vi "e.gate ASCII Write Value - CORE.vi"(6 "Value":dbl, 8 "error in (no error)":errorcluster, 9 "Boolean":bool=TRUE, 10 "Channel":i32, 11 "e.gate Configuration In":T1) -> (0 "error out":errorcluster, 3 "e.gate Configuration Out":T1)   [LabVIEW 2016]
doc: "<B>AMC - Analytik & Messtechnik GmbH Chemnitz</B>\n\nLabVIEW Drivers for e.gate / e.pac series from Gantner Instruments\n\nThis VI writes a value specified by <B>Channel</B> to a device specified by <B>connection ID In</B>."
uses:
  e.gate Configuration.ctl
  e.gate Channel Data.ctl
  e.gate Data Type.ctl
  e.gate Protocol Type.ctl
  e.gate Module  Data.ctl
  e.gateHSP_DLLhandle.ctl
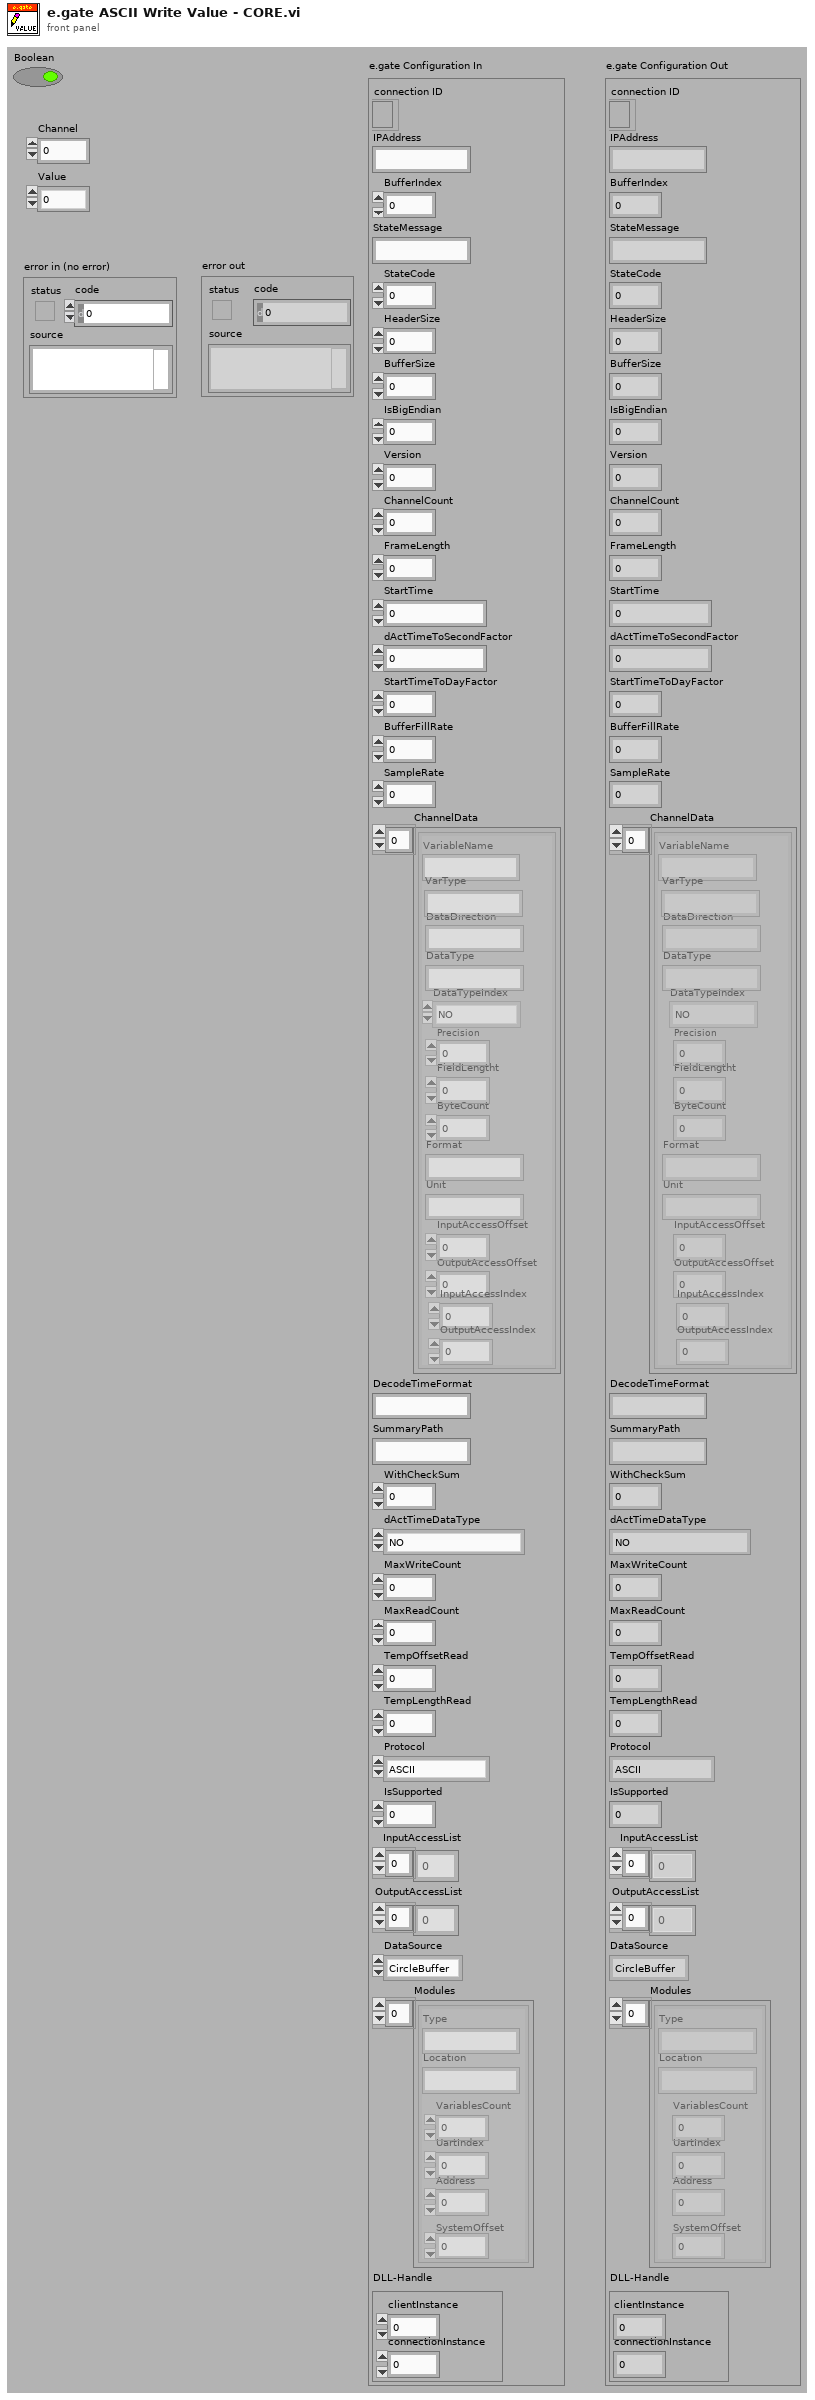
[diagram p1: front panel]
types:
  T1 = typedef "e.gate Configuration.ctl" = cluster{"connection ID":refnum<k5>, "IPAddress":string, "BufferIndex":i32, "StateMessage":string, "StateCode":i8, "HeaderSize":i32, "BufferSize":i32, "IsBigEndian":i32, "Version":i32, "ChannelCount":i32, "FrameLength":i32, "StartTime":dbl, "dActTimeToSecondFactor":dbl, "StartTimeToDayFactor":dbl, "BufferFillRate":dbl, "SampleRate":dbl, "ChannelData":T2[], "DecodeTimeFormat":string, "SummaryPath":string, "WithCheckSum":i32, "dActTimeDataType":T3, "MaxWriteCount":i32, "MaxReadCount":i32, "TempOffsetRead":i32, "TempLengthRead":i32, "Protocol":T4, "IsSupported":i32, "InputAccessList":i32[], "OutputAccessList":i32[], "DataSource":enum16{"CircleBuffer", "test.con Logger", "test.con Archive"}, "Modules":T5[], "DLL-Handle":T6}
  T2 = typedef "e.gate Channel Data.ctl" = cluster{"VariableName":string, "DataDirection":string, "DataType":string, "DataTypeIndex":T3, "Precision":i16, "FieldLengtht":i16, "ByteCount":i32, "Format":string, "Unit":string, "InputAccessOffset":i32, "OutputAccessOffset":i16, "InputAccessIndex":i16, "OutputAccessIndex":i16, "VarType":string}
  T3 = typedef "e.gate Data Type.ctl" = enum16{"NO", "BOOL", "SINT8", "USINT8", "SINT16", "USINT16", "SINT32", "USINT32", "FLOAT", "SET8", "SET16", "SET32", "DOUBLE", "SINT64", "USINT64", "SET64"}
  T4 = typedef "e.gate Protocol Type.ctl" = enum16{"ASCII", "HighspeedPort Online", "HighspeedPort Buffer", "eGateHighspeedPortDLL "}
  T5 = typedef "e.gate Module  Data.ctl" = cluster{"Type":string, "Location":string, "VariablesCount":i16, "UartIndex":i16, "Address":i16, "SystemOffset":i16}
  T6 = typedef "e.gateHSP_DLLhandle.ctl" = cluster{"clientInstance":i32, "connectionInstance":i32}
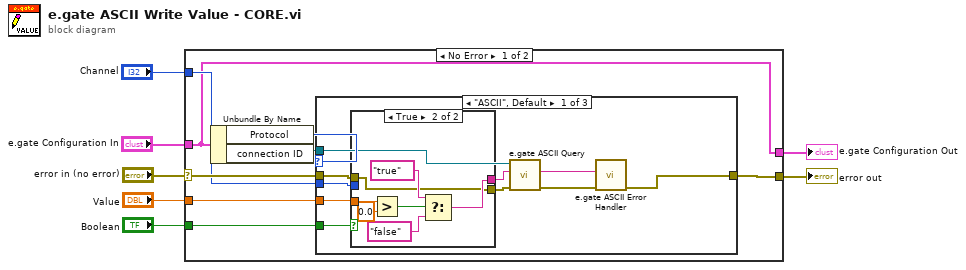
[diagram p0: block diagram]
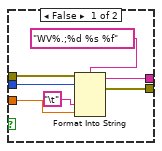
[diagram p2: hidden frame]
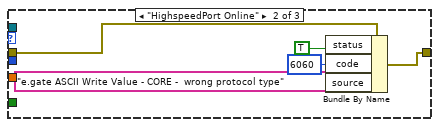
[diagram p3: hidden frame]
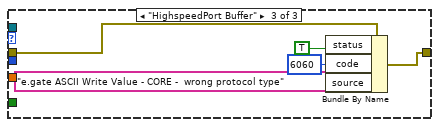
[diagram p4: hidden frame]
diagram:
  n1 = case shown="No Error" "error in (no error)" {
    selector: "error in (no error)" -> [w15 w51]
    tunnel: "e.gate Configuration In" -> [w10 w50]
    tunnel: "Channel" -> [w14 _]
    tunnel: [w10 w50] -> w4
    tunnel: [w12 w51] -> w3
    tunnel: "Value" -> [w13 _]
    tunnel: "Boolean" -> [w8 _]
    frame No Error {
      n2 = Unbundle By Name(w10) -> ("Protocol"=w9:T4, "connection ID"=w11:refnum<k5>)
      n3 = case shown="\"ASCII\", Default" w9 {
        tunnel: w15 -> [w25 w40 w45]
        tunnel: w14 -> [w24 _ _]
        tunnel: w13 -> [w18 _ _]
        tunnel: [w20 w41 w46] -> w12
        tunnel: w11 -> [w19 _ _]
        tunnel: w8 -> [w17 _ _]
        frame "ASCII", Default {
          n4 = case shown="True" w17 {
            tunnel: w25 -> [w32 w33]
            tunnel: w24 -> [w31 _]
            tunnel: [w27 w33] -> w23
            tunnel: w18 -> [w29 w39]
            tunnel: [w26 w34] -> w16
            frame False {
              n5 = Format Into String(format string="WV%.;%d %s %f", error in=w32, w31, "\t", w29) -> (resulting string=w26:string, error out=w27:errorcluster)  [unwired: 1 in]
            }
            frame True {
              n6 = Greater?(x=w39, y=0.0) -> (0:w37:bool)
              n7 = Select(t="true", s=w37, f="false") -> (s? t:f=w34:string)
            }
          }
          n8 = call "e.gate ASCII Query.vi"("error in (no error)"=w23, "Command"=w16, "connection ID In"=w19) -> ("error out"=w22:errorcluster, "Response"=w21:string)  [unwired: 7 out]
          n9 = call "e.gate ASCII Error Handler.vi"("error in (no error)"=w22, "String"=w21) -> ("error out"=w20:errorcluster)  [unwired: 9 out]
        }
        frame "HighspeedPort Online" {
          n10 = Bundle By Name(cluster=w40, "status"=TRUE, "code"=6060, "source"="e.gate ASCII Write Value - CORE -  wrong protocol type") -> (w41:errorcluster)
        }
        frame "HighspeedPort Buffer" {
          n11 = Bundle By Name(cluster=w45, "status"=TRUE, "code"=6060, "source"="e.gate ASCII Write Value - CORE -  wrong protocol type") -> (w46:errorcluster)
        }
      }
    }
    frame Error {
    }
  }
  "error out" <- w3
  "e.gate Configuration Out" <- w4
